vi "moveInTreeCtrl.vi"(6 "Position":i32, 8 "error in (no error)":errorcluster, 9 "subNode tag":string, 10 "superNode tag":string, 11 "xceRootNode in":refnum<class "xceRootNode.lvclass">) -> (0 "error out":errorcluster, 3 "xceRootNode out":refnum<class "xceRootNode.lvclass">)   [LabVIEW 2013, in "xceRootNode.lvclass"]
uses:
  xceRootNode.lvclass
  xceRootNode.lvclass/xceRootNode.ctl
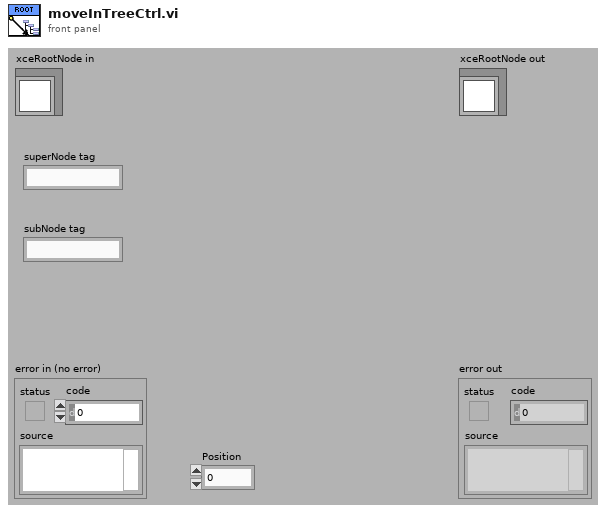
[diagram p1: front panel]
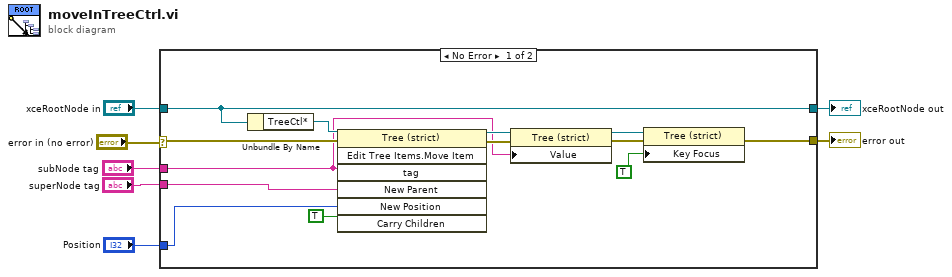
[diagram p0: block diagram]
diagram:
  n1 = case shown="No Error" "error in (no error)" {
    selector: "error in (no error)" -> [w16 w22]
    tunnel: [w9 w22] -> w6
    tunnel: [w20 w21] -> w4
    tunnel: "xceRootNode in" -> [w20 w21]
    tunnel: "subNode tag" -> [w12 _]
    tunnel: "superNode tag" -> [w18 _]
    tunnel: "Position" -> [w15 _]
    frame No Error {
      n2 = Unbundle By Name(w20) -> ("TreeCtl*"=w19:refnum<vi>)
      n3 = invoke class="Tree (strict)" method="Edit Tree Items.Move Item"(reference=w19, error in=w16, "tag"=w12, "New Parent"=w18, "New Position"=w15, "Carry Children"=TRUE ("Carry Children?")) -> (reference out=w14:refnum<vi>, error out=w13:errorcluster)  [unwired: 1 in, 5 out]
      n4 = property class="Tree (strict)"(reference=w14, error in=w13, "Value"=w12) -> (reference out=w11:refnum<vi>, error out=w10:errorcluster)
      n5 = property class="Tree (strict)"(reference=w11, error in=w10, "Key Focus"=TRUE) -> (error out=w9:errorcluster)  [unwired: 1 out]
    }
    frame Error {
    }
  }
  "error out" <- w6
  "xceRootNode out" <- w4
